vi "log_template.vi"(9 "接收报文":string, 11 "发送报文":string) -> ()   [LabVIEW 2015]
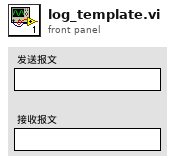
[diagram p1: front panel]
types:
  T1 = enum16{"open", "replace", "create", "open or create", "replace or create", "replace or create with confirmation"}
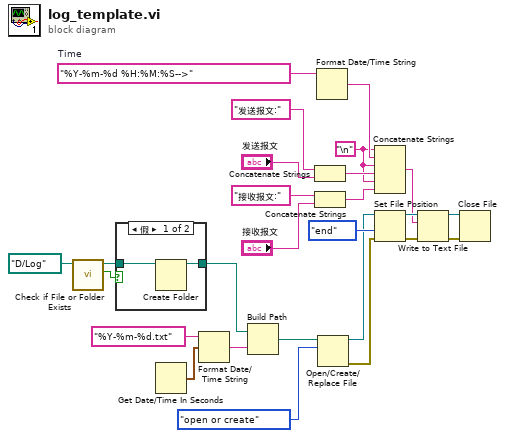
[diagram p0: block diagram]
diagram:
  w3 = "\n"
  w18 = "%Y-%m-%d %H:%M:%S-->"  # Time
  n1 = call <vilib>:"Check if File or Folder Exists.vi"("path"=path "D:/Log" ("路径")) -> ("file or folder exists?"=w24:bool, "dup path"=w25:path)  [unwired: 8 in, 1 out]
  n2 = case shown="假" w24 {
    tunnel: w25 -> [w28 w29]
    tunnel: [w27 w29] -> w22
    frame False {
      n3 = Create Folder(path (use dialog)=w28) -> (created path=w27:path)  [unwired: 2 in, 2 out]
    }
    frame True {
    }
  }
  n4 = Get Date/Time In Seconds() -> (seconds since 1Jan1904=w20:timestamp)
  n5 = Format Date/Time String(time format string (%c)="%Y-%m-%d.txt" ("时间格式字符串(%c)"), seconds (now)=w20) -> (date/time string=w19:string)  [unwired: 1 in]
  n6 = Build Path(base path=w22, name or relative path=w19) -> (appended path=w26:path)
  n7 = Concatenate Strings("发送报文:", "发送报文") -> (w6:string)
  n8 = Concatenate Strings("接收报文:", "接收报文") -> (w2:string)
  n9 = Format Date/Time String(time format string (%c)=w18) -> (date/time string=w9:string)  [unwired: 2 in]
  n10 = Open/Create/Replace File(file path (use dialog)=w26, operation (0:open)=T1."open or create" ("操作(0:open)")) -> (refnum out=w13:refnum<file>, error out=w14:errorcluster)  [unwired: 4 in, 1 out]
  n11 = Concatenate Strings(w3, w9, w3, w6, w3, w2) -> (w1:string)
  n12 = Set File Position(refnum=w13, from (0:start)=enum16{"start", "end", "current"}."end" ("自（0:起始）"), error in=w14) -> (refnum out=w15:refnum<file>, error out=w16:errorcluster)  [unwired: 1 in]
  n13 = Write to Text File(file (use dialog)=w15, text=w1, error in=w16) -> (refnum out=w12:refnum<file>, error out=w11:errorcluster)  [unwired: 1 in, 1 out]
  n14 = Close File(refnum=w12, error in=w11) -> ()  [unwired: 2 out]
